vi "Get AI.vi"(0 "Module Ref":refnum<class "Modbus Master.lvclass">, 11 "error in (no error)":errorcluster) -> (4 "Modbus master out":refnum<class "Modbus Master.lvclass">, 6 "AI Measurment":u16[](array[numeric]), 15 "error out":errorcluster)   [LabVIEW 2024]
doc: "Read back analogue input registers"
uses:
  <vilib>/NI/Modbus Library/API/Master/Modbus Master.lvclass
panel:
  # "Channel 0"
  # "Channel 1"
  # "Channel 2"
  # "Channel 3"
  # "Channel 4"
  # "Channel 5"
  # "Channel 6"
  # "Channel 7"
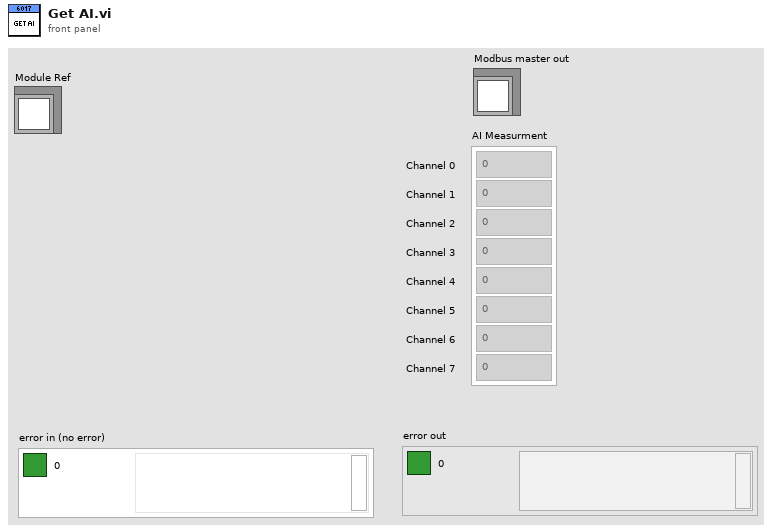
[diagram p1: front panel]
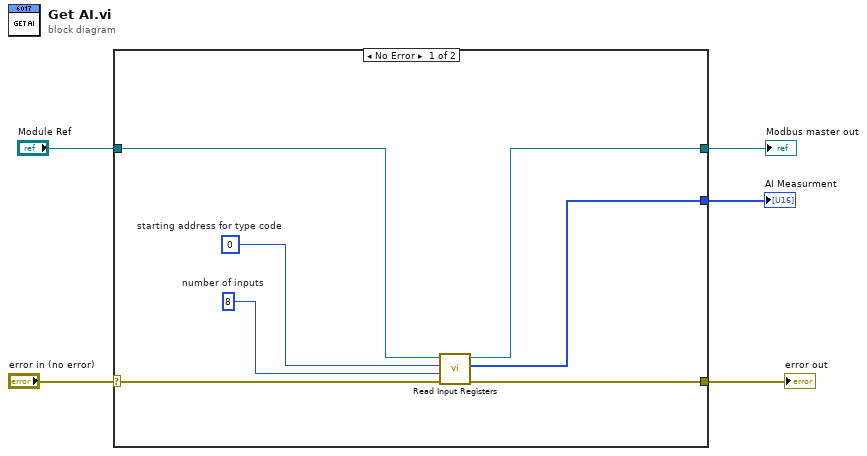
[diagram p0: block diagram]
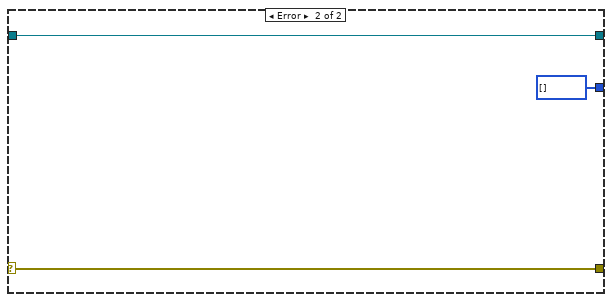
[diagram p2: hidden frame]
diagram:
  n1 = case shown="No Error" "error in (no error)" {
    selector: "error in (no error)" -> [w12 w14]
    tunnel: "Module Ref" -> [w9 w15]
    tunnel: [w11 w14] -> w3
    tunnel: [w10 w15] -> w2
    tunnel: [w6 u16[] [] ("register values")] -> w1
    frame No Error {
      w7 = u16 8  # number of inputs
      w8 = u16 0  # starting address for type code
      n2 = call-dynamic "Read Input Registers.vi"("error in"=w12, "number of inputs"=w7, "starting address"=w8, "Modbus master in"=w9) -> ("error out"=w11:errorcluster, "register values"=w6:u16[], "Modbus master out"=w10:refnum<class "Modbus Master.lvclass">)  [unwired: 5 in]
    }
    frame Error {
    }
  }
  "error out" <- w3
  "Modbus master out" <- w2
  "AI Measurment" <- w1
